vi "GetResponse.vi"(0 "Response First Line + CRLF":string="HTTP/1.1 200 OK\r\n", 2 "Response Header Template":string="User-Agent: LabVIEW WebServer/0.1\nDate: RESPONSE_DATE\nExpires: RESPONSE_DATE\nIgnore-Buffer: xXxBUFFERxXx\nContent-Type: CONTENT_TYPE\nContent-Length: RESPONSE_LENGTH\nConnection: keep-alive", 3 "Content Type":string, 4 "ResponseBody":string) -> (5 "TotalResponseOut":string)   [LabVIEW 2014]
doc: "Compiles the response from the serveri"
panel:
  out "TotalResponseOutLength":i32
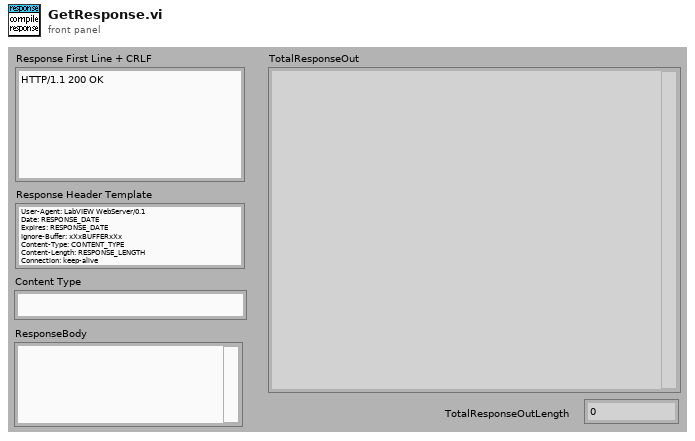
[diagram p1: front panel]
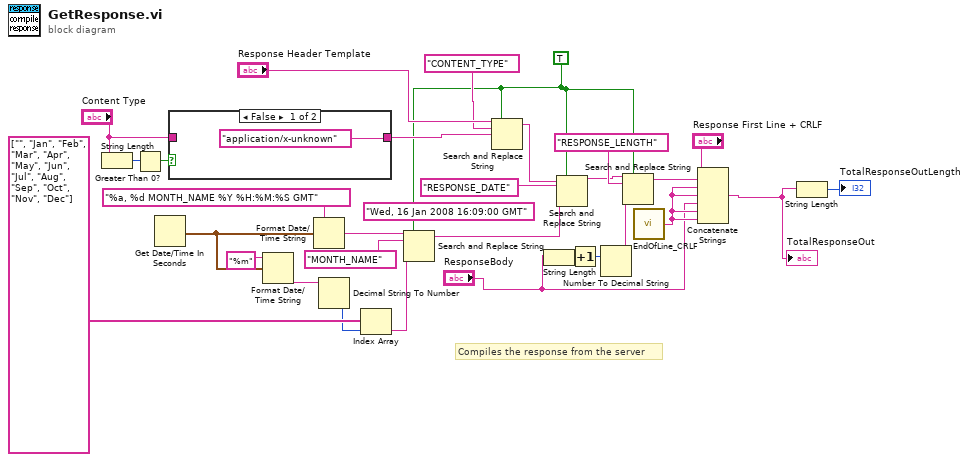
[diagram p0: block diagram]
diagram:
  w7 = TRUE ("replace all? (F)")
  (unwired) "Wed, 16 Jan 2008 16:09:00 GMT" ("replace string (\"\")")
  # "Compiles the response from the server"
  n1 = String Length(string="Content Type") -> (length=w20:i32)
  n2 = Greater Than 0?(x=w20) -> (x > 0?=w21:bool)
  n3 = Get Date/Time In Seconds() -> (seconds since 1Jan1904=w16:timestamp)
  n4 = case shown="False" w21 {
    tunnel: "Content Type" -> [_ w32]
    tunnel: ["application/x-unknown" w32] -> w18
    frame False {
    }
    frame True {
    }
  }
  n5 = Format Date/Time String(time format string (%c)="%m", seconds (now)=w16) -> (date/time string=w14:string)  [unwired: 1 in]
  n6 = Format Date/Time String(time format string (%c)="%a, %d MONTH_NAME %Y %H:%M:%S GMT", seconds (now)=w16) -> (date/time string=w11:string)  [unwired: 1 in]
  n7 = Decimal String To Number(string=w14) -> (number=w12:i32)  [unwired: 3 out]
  n8 = Index Array(array=string[] ["", "Jan", "Feb", "Mar", "Apr", "May", "Jun", "Jul", "Aug", "Sep", "Oct", "Nov", "Dec"], index=w12) -> (element=w9:string)
  n9 = Search and Replace String(replace all?=w7, input string=w11, search string="MONTH_NAME", replace string=w9) -> (result string=w8:string)  [unwired: 4 in, 3 out]
  n10 = Search and Replace String(replace all?=w7, input string="Response Header Template", search string="CONTENT_TYPE", replace string=w18) -> (result string=w28:string)  [unwired: 4 in, 3 out]
  n11 = String Length(string="ResponseBody") -> (length=w3:i32)
  n12 = Search and Replace String(replace all?=w7, input string=w28, search string="RESPONSE_DATE", replace string=w8) -> (result string=w23:string)  [unwired: 4 in, 3 out]
  n13 = Increment(x=w3) -> (x+1=w2:i32)
  n14 = Number To Decimal String(number=w2) -> (decimal integer string=w25:string)  [unwired: 1 out]
  n15 = Search and Replace String(replace all?=w7, input string=w23, search string="RESPONSE_LENGTH", replace string=w25) -> (result string=w26:string)  [unwired: 4 in, 3 out]
  n16 = call <userlib>:"EndOfLine_CRLF.vi"() -> ("String"=w6:string)
  n17 = Concatenate Strings("Response First Line + CRLF", w26, w6, w6, "ResponseBody", w6, w6) -> (w4:string)
  "TotalResponseOut" <- w4
  n18 = String Length(string=w4) -> (length=→"TotalResponseOutLength":i32)
